vi "Wait for State.vi"(5 "timeout (ms)":u32=5000, 8 "error in (no error)":errorcluster, 9 "stream state":T1, 10 "stream index":i32, 11 "refnum in":refnum<k20>) -> (0 "error out":errorcluster, 3 "refnum out":refnum<k20>)   [LabVIEW 2015, in "niInstr Streaming v1 Host.lvlib"]
doc: "This VI is used internally to hold execution until the specified state is reached.\n\n<B>Input Parameters</B>\n\n<B>error in (no error)</B> 'error in' can accept error information wired from VIs previously called. Use this information to decide if any functionality should be bypassed in the event of errors from other VIs.\n\nRight-click the 'error in' control on the front panel and select 'Explain Error' or 'Explain Warning' from the shortcut menu for more information about the error.\n\n<B>stream state</B> The VI will wait until this state is reached.\n\n<B>stream index</B> Selects which stream index this VI will interface to. This is the index number at the end of the host interface controls (0..7).\n\n<B>refnum in</B> Wire in the session obtained from Open FPGA Reference.\n\n<B>Output Parameters</B>\n\n<B>error out</B> contains error information. This output provides standard error out functionality."
uses:
  <instrlib>/_niInstr/Streaming/v1/Host/niInstr Streaming v1 Host.lvlib
  <instrlib>/_niInstr/Streaming/v1/Common/Stream State.ctl
  <vilib>/Utility/error.llb/Error Cluster From Error Code.vi
  <vilib>/ErrorRing/Error Ring.xnode
  <instrlib>/_niInstr/Streaming/v1/Common/niInstr Streaming v1 Common.lvlib
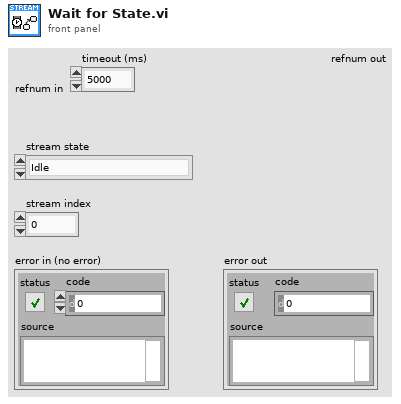
[diagram p1: front panel]
types:
  T1 = typedef "niInstr Streaming v1 Common.lvlib/Stream State.ctl" = enum8{"Idle", "Finite Transfer", "Continuous", "Done", "Error", "Not Ready", "Cancel"}
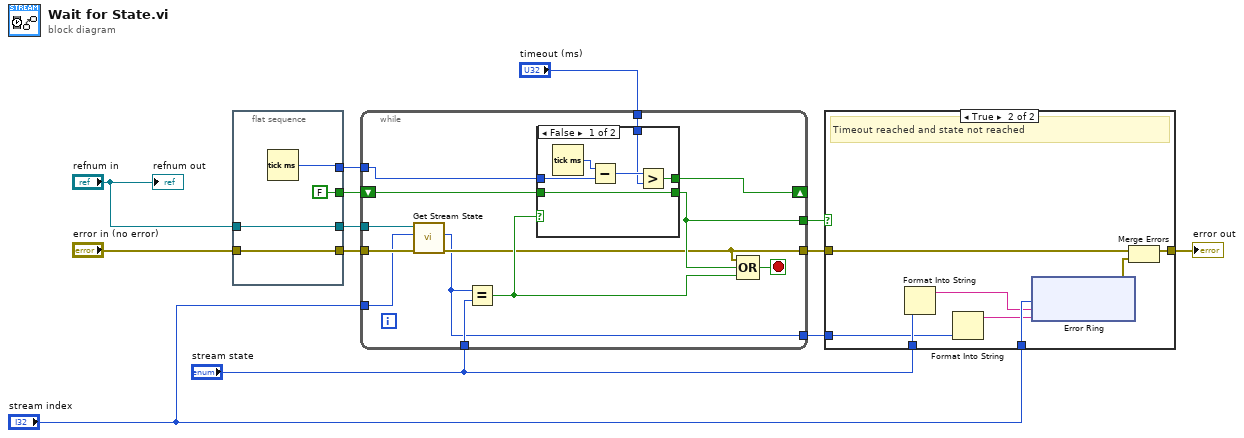
[diagram p0: block diagram]
diagram:
  n1 = flat-sequence {
    tunnel: [w14] -> w4
    tunnel: [FALSE] -> w8
    tunnel: [w16] -> w9
    tunnel: "error in (no error)" -> [w16]
    tunnel: "refnum in" -> [w15]
    tunnel: [w15] -> w12
    frame #0 {
      n2 = Tick Count (ms)() -> (millisecond timer value=w14:u32)
    }
  }
  n3 = while {
    tunnel: w12 -> [w28]
    tunnel: w9 -> [w29]
    tunnel: w4 -> [w25]
    tunnel: [w21] -> w5
    tunnel: "stream index" -> [w27]
    shift-right: [w24] -> _
    shift-left: w8 -> [w23]
    tunnel: [w22] -> w13
    tunnel: "stream state" -> [w20]
    tunnel: "timeout (ms)" -> [w19]
    tunnel: [w18] -> w1
    stop <- w30 stop-if-true
    n4 = call <instrlib>:"Get Stream State.vi"("error in (no error)"=w29, "stream index"=w27, "refnum in"=w28) -> ("error out"=w21:errorcluster, "stream state"=w18:T1)  [unwired: 6 in, 1 out]
    n5 = Equal?(x=w18, y=w20) -> (x = y?=w26:bool)
    n6 = case shown="False" w26 {
      tunnel: w25 -> [w34 _]
      tunnel: [w33 _] -> w24
      tunnel: w23 -> [w32 _]
      tunnel: [w32 _] -> w22
      tunnel: w19 -> [w31 _]
      frame False {
        n7 = Tick Count (ms)() -> (millisecond timer value=w35:u32)
        n8 = Subtract(x=w35, y=w34) -> (x-y=w36:u32)
        n9 = Greater?(x=w36, y=w31) -> (0:w33:bool)
      }
      frame True {
      }
    }
    n10 = Compound Arithmetic op=OR(w21, w22, w26) -> (w30:bool)
  }
  n11 = case shown="True" w13 {
    tunnel: w5 -> [w37 w45]
    tunnel: [w37 w44] -> w6
    tunnel: "stream index" -> [_ w43]
    tunnel: "stream state" -> [_ w41]
    tunnel: w1 -> [_ w39]
    frame False {
    }
    frame True {
      # "Timeout reached and state not reached"
      n12 = Format Into String(w41) -> (resulting string=w40:string)  [unwired: 3 in, 1 out]
      n13 = Format Into String(w39) -> (resulting string=w38:string)  [unwired: 3 in, 1 out]
      n14 = xnode "Error Ring"("parameter 0"=w43, "parameter 1"=w40, "parameter 2"=w38) -> ("error out"=w42:errorcluster)
      n15 = Merge Errors(w45, w42) -> (w44:errorcluster)
    }
  }
  "error out" <- w6
  "refnum out" <- "refnum in"
